vi "zmq_disconnect.vi"(3 "error in":errorcluster, 4 "endpoint":string, 5 "socket in":refnum<class "zmq_socket.lvclass">) -> (0 "error out":errorcluster, 2 "socket out":refnum<class "zmq_socket.lvclass">)   [LabVIEW 2019, in "zeromq.lvlib" / "zmq_socket.lvclass"]
doc: "Disconnect the given socket from the specified <b>endpoint</b>. Opposite of zmq_connect. Use zmq_close to disconnect from all endpoints.\n\nDetailed API documentation: http://api.zeromq.org/3-2:zmq-disconnect"
uses:
  zmq_socket.lvclass
  zmq_socket.lvclass/zmq_socket.ctl
  <vilib>/Utility/error.llb/Error Cluster From Error Code.vi
  zeromq.lvlib
panel:
  # "ØMQ"
  # "labview"
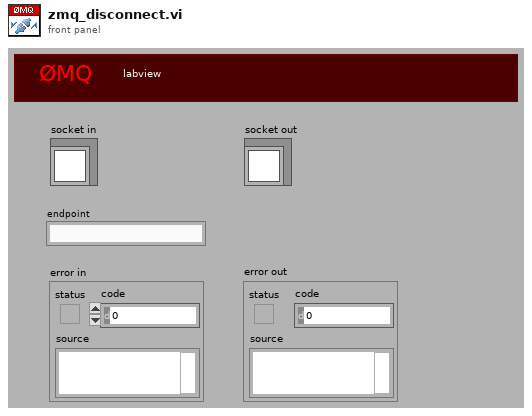
[diagram p1: front panel]
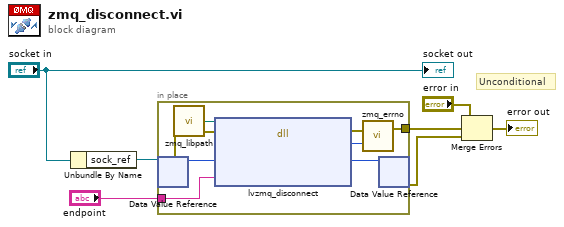
[diagram p0: block diagram]
diagram:
  # "Unconditional"
  n1 = Unbundle By Name("socket in") -> ("sock_ref"=w4:refnum<data-value>)
  n2 = in-place {
    in-place-border: "endpoint" -> [w15]
    in-place-border: [w12] -> w6
    n3 = in-place-dvr #1(w4) -> (w11:u64, w8:errorcluster)
    n4 = call "zmq_libpath.vi"() -> ("path"=w9:path)
    n5 = dll-call lib="?" fn="lvzmq_disconnect" ("zmq_labview.dll:lvzmq_connect")(path in=w9, error in=w8, "sock_obj"=w11, "endpoint"=w15) -> (error out=w14:errorcluster, "return type"=w13:i32, "sock_obj"=w10:u64)  [unwired: 2 in, 1 out]
    n6 = call "zmq_errno.vi"("retval"=w13, "error in"=w14) -> ("error out"=w12:errorcluster)  [unwired: 1 out]
    n7 = in-place-dvr #1(w10) -> (w1:errorcluster)  [unwired: 1 out]
  }
  n8 = Merge Errors("error in", w6, w1) -> (→"error out":errorcluster)
  "socket out" <- "socket in"
